vi "TrimQuotes.vi"(10 "With \"":string) -> (2 "Without \"":string)   [LabVIEW 2020]
uses:
  <vilib>/regexp/Match Regular Expression.xnode
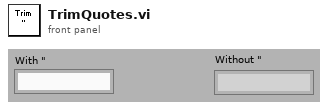
[diagram p1: front panel]
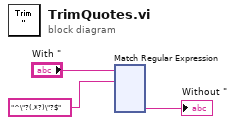
[diagram p0: block diagram]
diagram:
  n1 = xnode "Match Regular Expression"("input string"="With \"", "regular expression"="^\"?(.*?)\"?$") -> ("submatch 1"=→"Without \"":string)  [unwired: 4 in, 5 out]
